vi "read config.vi"(8 "error in (no error)":errorcluster, 10 "Path":path=path "C:/Users/grove/Desktop/LabVIEW/Git/dqmh-lvoop-template/Config/dqmh-lvoop-template/uno-config.json", 11 "Arduino Uno in":refnum<class "Arduino Uno.lvclass">) -> (0 "error out":errorcluster, 3 "Arduino Uno out":refnum<class "Arduino Uno.lvclass">)   [LabVIEW 2025, in "USB IO.lvlib" / "Arduino Uno.lvclass"]
uses:
  Arduino Uno.lvclass
  Arduino Uno.lvclass/Arduino Uno.ctl
  5079893e-9f81-444c-b477-d8ba1a1882ba.vi
  <vilib>/JDP Science/JSONtext/JSON text to Variant.vi
  <vilib>/JDP Science/JSONtext/LVClass Serializer/JSONtext LVClass Serializer.lvclass
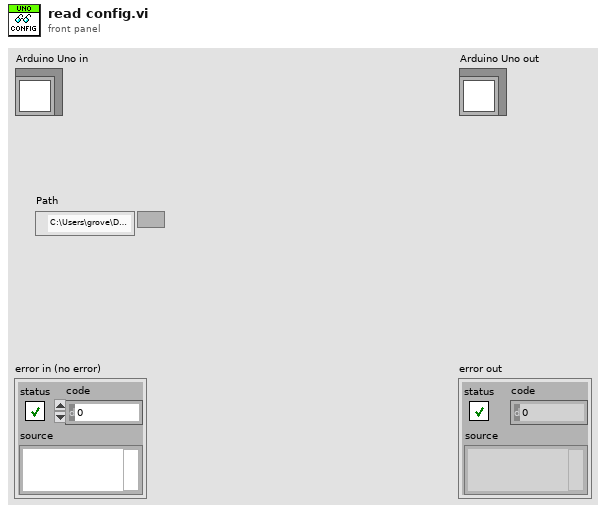
[diagram p1: front panel]
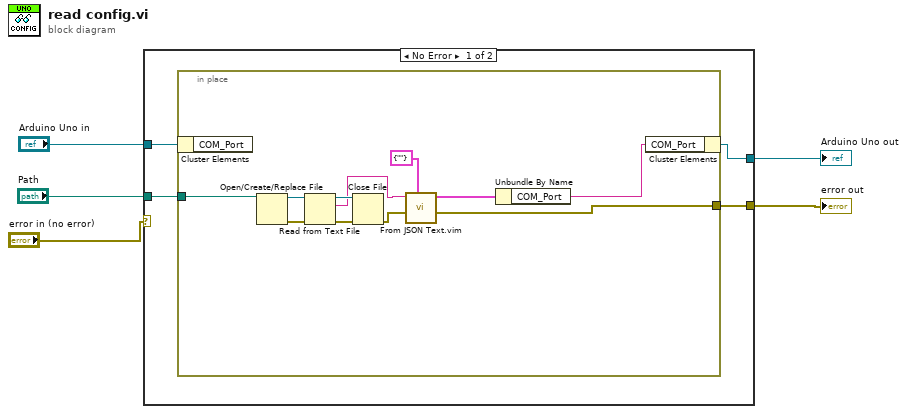
[diagram p0: block diagram]
diagram:
  n1 = case shown="No Error" "error in (no error)" {
    selector: "error in (no error)" -> [_ w22]
    tunnel: [w6 w22] -> w4
    tunnel: "Arduino Uno in" -> [w9 w21]
    tunnel: [w8 w21] -> w2
    tunnel: "Path" -> [w7 _]
    frame No Error {
      n2 = in-place {
        in-place-border: w7 -> [w20]
        in-place-border: [w10] -> w6
        n3 = in-place-cluster #1(w9) -> ()  [unwired: 1 out]
        n4 = Open/Create/Replace File(file path (use dialog)=w20) -> (refnum out=w18:refnum<file>, error out=w19:errorcluster)  [unwired: 5 in, 1 out]
        n5 = Read from Text File(file (use dialog)=w18, error in=w19) -> (refnum out=w16:refnum<file>, text=w15:string, error out=w17:errorcluster)  [unwired: 2 in, 1 out]
        n6 = Close File(refnum=w16, error in=w17) -> (error out=w11:errorcluster)  [unwired: 1 out]
        n7 = call "From JSON Text.vim"("Data Type and Default Value"=cluster{"COM_Port":string} {"COM_Port"=""}, "error in (no error)"=w11, "JSON"=w15) -> ("error out"=w10:errorcluster, "Data out"=w13:cluster{"COM_Port":string})  [unwired: 7 in]
        n8 = Unbundle By Name(w13) -> ("COM_Port"=w12:string)
        n9 = in-place-cluster #1("COM_Port"=w12) -> (w8:refnum<class "Arduino Uno.lvclass">)
      }
    }
    frame Error {
    }
  }
  "error out" <- w4
  "Arduino Uno out" <- w2
